vi "transmitter_labviewPID.vi"() -> ()   [LabVIEW 2025]
uses:
  <vilib>/Instr/_visa.llb/VISA Configure Serial Port (Instr).vi
panel:
  in  "timeout (10sec)":u32=10000
  out "output string":string
  out "Raw string":string
  in  "Reverse":bool
  in  "Forward":bool
  out "Temperature":string
  out "Motor Level":string
  out "LDR Level":string
  out "Humidity":string
  out "Motor feedback":i32(graph)
  in  "Start PID":bool
  in  "Setpoint (PWM)":u8 max=100 step=5
  in  "stop bits (10: 1 bit)":u16(ring)=10 items=["1.0"=10, "1.5"=15, "2.0"=20]
  in  "parity (0:none)":enum16{"None", "Odd", "Even", "Mark", "Space"}(ring)
  in  "data bits (8)":u16=8 min=5 max=8 step=1
  in  "baud rate (9600)":u32=9600
  in  "?":bool
  in  "Stop":bool
  in  "VISA resource COM PORT":refnum<visa-resource-name>
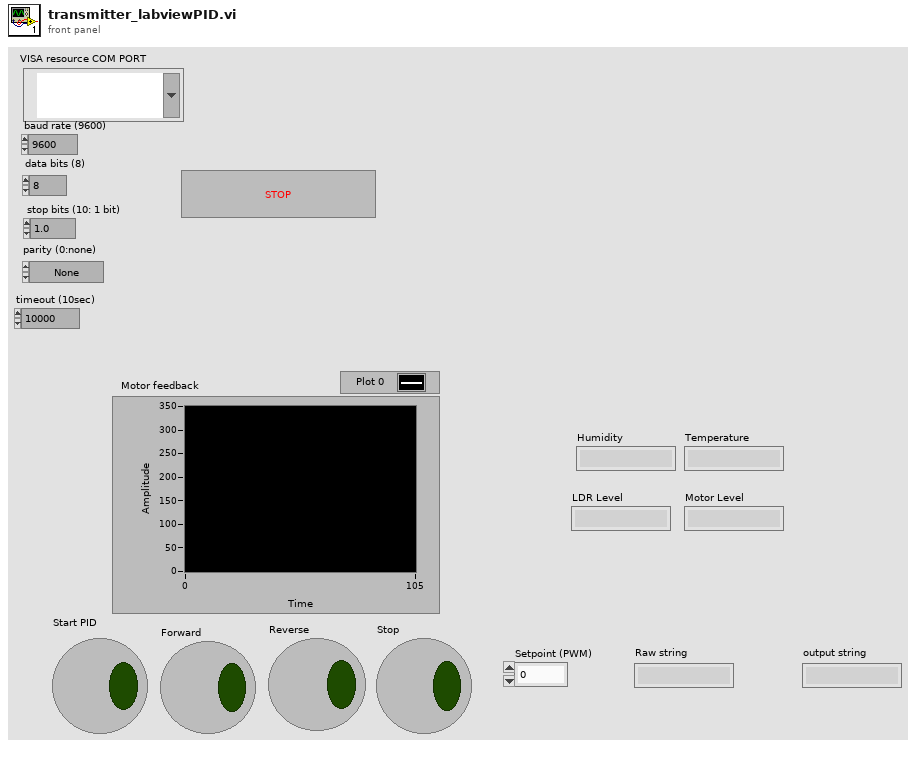
[diagram p1: front panel]
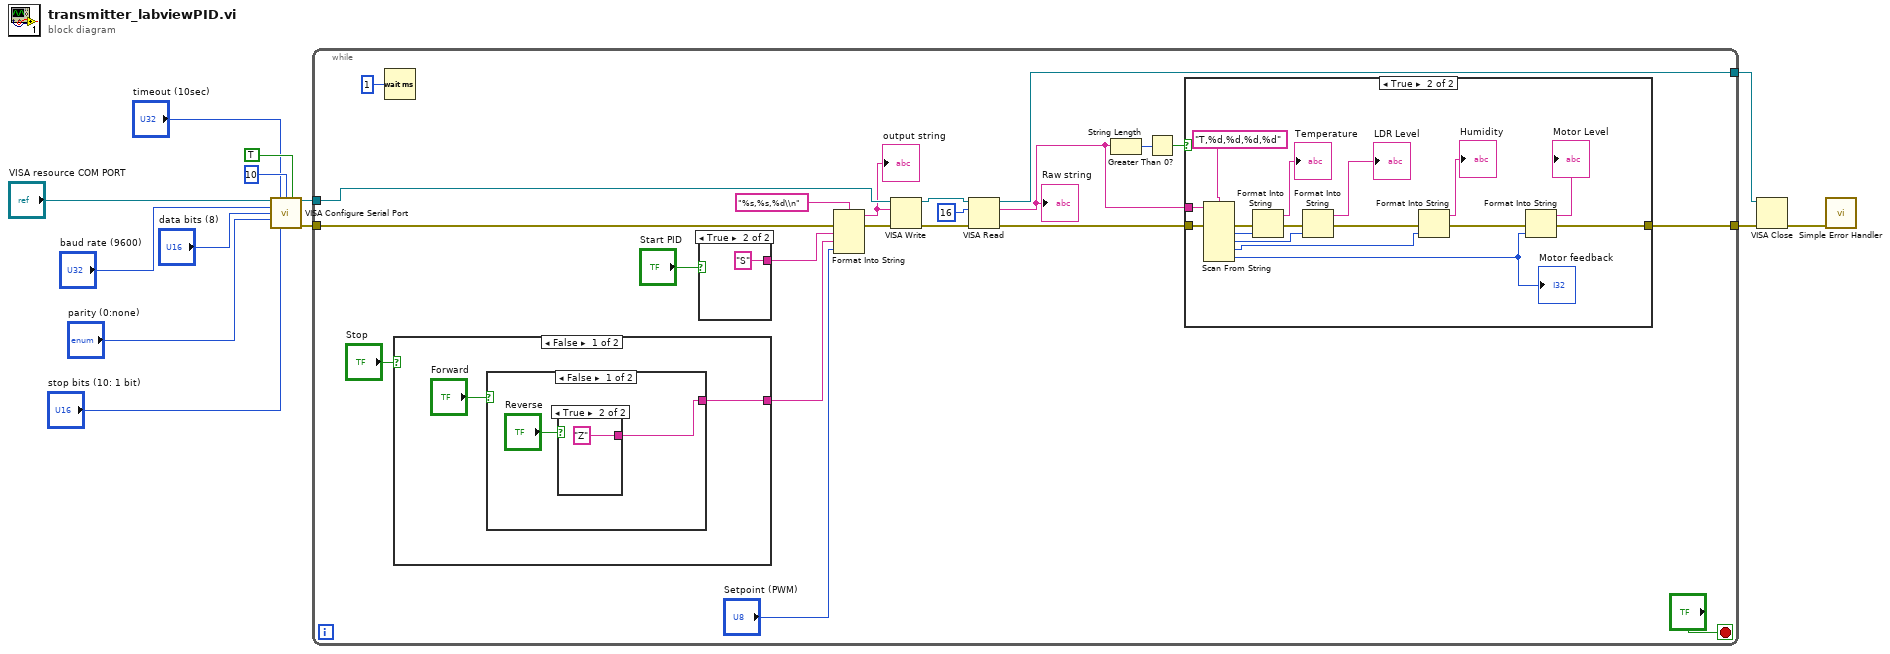
[diagram p0: block diagram]
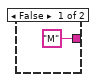
[diagram p3: hidden frame]
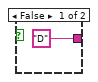
[diagram p4: hidden frame]
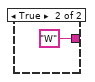
[diagram p5: hidden frame]
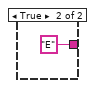
[diagram p6: hidden frame]
diagram:
  n1 = call-poly "VISA Configure Serial Port"("VISA resource name"="VISA resource COM PORT", "timeout (10sec)"="timeout (10sec)", "termination char\n(0xA = '\\n' = LF)"=u8 10 ("termination char\n(0xA = '\\n' = LF)"), "Enable Termination\nChar (T)"=TRUE ("Enable Termination\nChar (T)"), "baud rate (9600)"="baud rate (9600)", "data bits (8)"="data bits (8)", "parity (0:none)"="parity (0:none)", "stop bits (10: 1 bit)"="stop bits (10: 1 bit)") -> ("VISA resource name out"=w7:refnum<visa-resource-name>, "error out"=w6:errorcluster)  [unwired: 6 in]
  n2 = while {
    tunnel: w6 -> [w15]
    tunnel: w7 -> [w22]
    tunnel: [w29] -> w4
    tunnel: [w16] -> w3
    stop <- "?" stop-if-true
    n3 = Wait (ms)(milliseconds to wait=u32 1 ("millisecond timer value")) -> ()  [unwired: 1 out]
    n4 = case shown="False" "Stop" {
      tunnel: [w54 "E" ("write buffer")] -> w24
      frame False {
        n5 = case shown="False" "Forward" {
          tunnel: [w56 "W" ("write buffer")] -> w54
          frame False {
            n6 = case shown="True" "Reverse" {
              tunnel: ["D" ("write buffer") "Z" ("write buffer")] -> w56
              frame False {
              }
              frame True {
              }
            }
          }
          frame True {
          }
        }
      }
      frame True {
      }
    }
    n7 = case shown="True" "Start PID" {
      tunnel: ["M" ("write buffer") "S" ("write buffer")] -> w25
      frame False {
      }
      frame True {
      }
    }
    n8 = Format Into String(format string="%s,%s,%d\\n", error in=w15, w25, w24, "Setpoint (PWM)") -> (resulting string=w18:string, error out=w14:errorcluster)  [unwired: 1 in]
    "output string" <- w18
    n9 = VISA Write(VISA resource name=w22, write buffer=w18, error in (no error)=w14) -> (VISA resource name out=w28:refnum<visa-resource-name>, error out=w27:errorcluster)  [unwired: 1 out]
    n10 = VISA Read(VISA resource name=w28, byte count=u32 16, error in (no error)=w27) -> (VISA resource name out=w29:refnum<visa-resource-name>, read buffer=w19:string, error out=w17:errorcluster)  [unwired: 1 out]
    "Raw string" <- w19
    n11 = String Length(string=w19) -> (length=w20:i32)
    n12 = Greater Than 0?(x=w20) -> (x > 0?=w21:bool)
    n13 = case shown="True" w21 {
      tunnel: w19 -> [_ w43]
      tunnel: w17 -> [w35 w42]
      tunnel: [w35 w37] -> w16
      frame False {
      }
      frame True {
        n14 = Scan From String(format string="T,%d,%d,%d,%d", input string=w43, error in=w42) -> (error out=w41:errorcluster, output 1=w48:i32, output 2=w49:i32, output 3=w50:i32, output 4=w51:i32)  [unwired: 5 in, 2 out]
        "Motor feedback" <- w51
        n15 = Format Into String(error in=w41, w48) -> (resulting string=→"Temperature":string, error out=w40:errorcluster)  [unwired: 2 in]
        n16 = Format Into String(error in=w40, w49) -> (resulting string=→"LDR Level":string, error out=w39:errorcluster)  [unwired: 2 in]
        n17 = Format Into String(error in=w39, w50) -> (resulting string=→"Humidity":string, error out=w38:errorcluster)  [unwired: 2 in]
        n18 = Format Into String(error in=w38, w51) -> (resulting string=→"Motor Level":string, error out=w37:errorcluster)  [unwired: 2 in]
      }
    }
  }
  n19 = VISA Close(VISA resource name=w4, error in (no error)=w3) -> (error out=w5:errorcluster)
  n20 = call <vilib>:"Simple Error Handler.vi"("error in (no error)"=w5) -> ()  [unwired: 4 in, 5 out]
